vi "Rawdata_Viewer.vi"() -> ()   [LabVIEW 2020]
uses:
  ctl/Image_RAW_Bayer_Pattern.ctl
  ctl/Image_Configuration.ctl
panel:
  out "Total Frame Num":i64
  in  "stop":bool
  in  "Display":bool
  in  "Frame Index":u32
  out "Image":T1(plugin-control)
  in  "Image Configuration":T2={"Width"=3840, "Height"=2160}
  in  "Bayer Pattern":T3=enum."RGGB (GRBG)"
  in  "RAWdata File Path":path
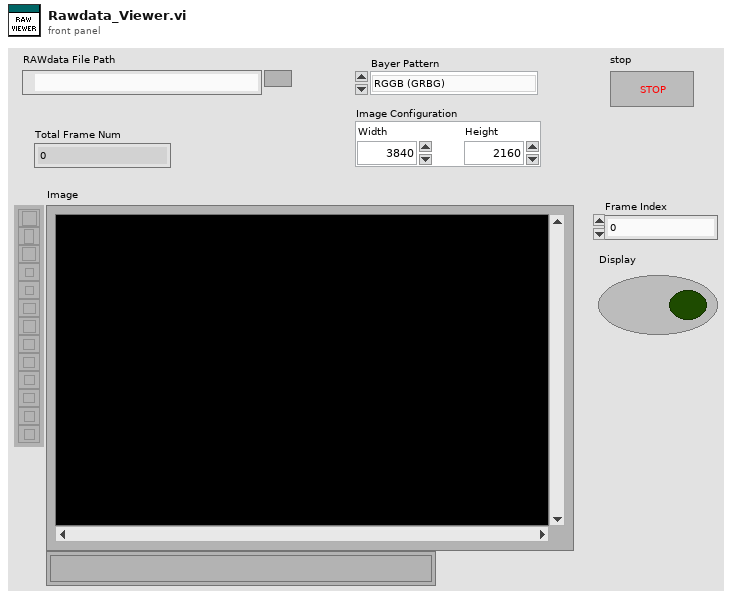
[diagram p1: front panel]
types:
  T1 = typedef "IMAQ Image.ctl" = refnum<image>
  T2 = typedef "Image_Configuration.ctl" = cluster{"Width":i32, "Height":i32}
  T3 = typedef "Image_RAW_Bayer_Pattern.ctl" = enum16{"GBRG (BGGR)", "GRBG (RGGB)", "BGGR (GBRG)", "RGGB (GRBG)", "CRBC (RCCB)"}
  T4 = typedef "Image_Data_Config.ctl" = cluster{"Lines of Image Data":u16, "Bytes per Even Line":u16, "Bytes per Odd Line":u16, "Image Data Type":u8, "Total Image Data Block Size":u32, "Image Data Block Offset":u32}
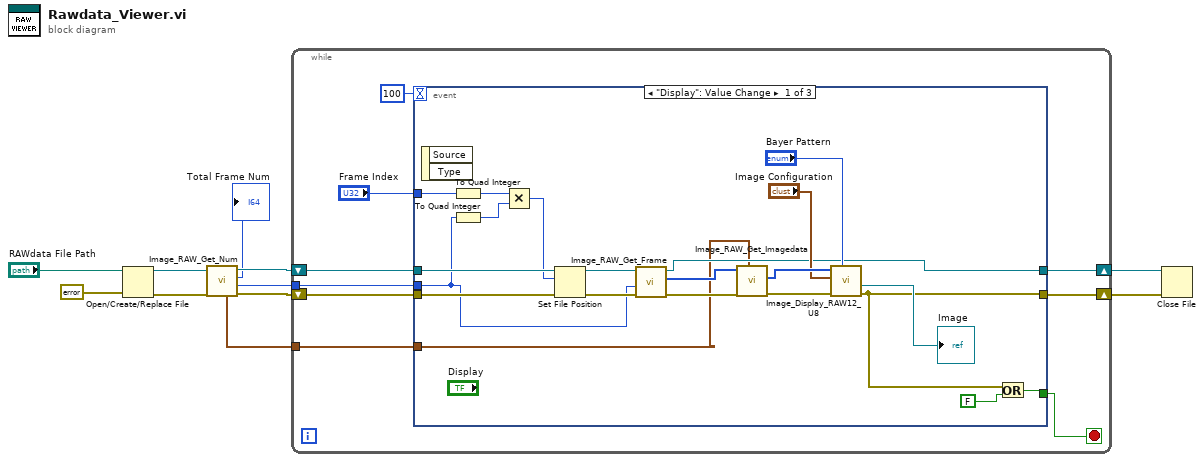
[diagram p0: block diagram]
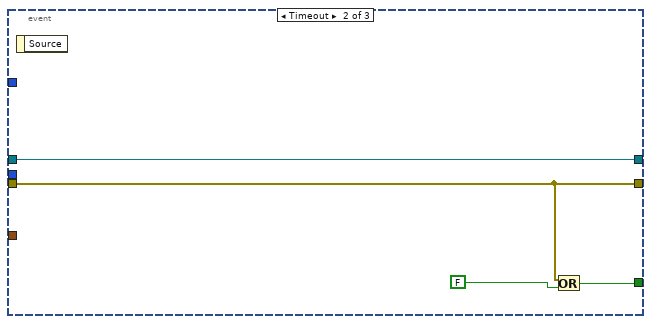
[diagram p2: hidden frame]
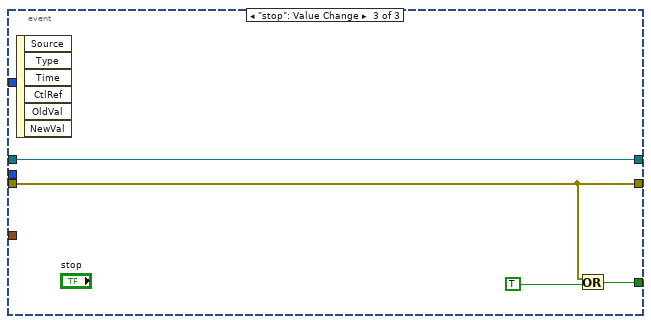
[diagram p3: hidden frame]
diagram:
  n1 = Open/Create/Replace File(file path (use dialog)="RAWdata File Path", error in=errorcluster {"status"=FALSE, "code"=0, "source"=""}) -> (refnum out=w10:refnum<file>, error out=w9:errorcluster)  [unwired: 4 in, 1 out]
  n2 = call "Image_RAW_Get_Num.vi"("error in (no error)"=w9, "RAW refnum In"=w10) -> ("error out"=w5:errorcluster, "Bytes per Frame"=w2:u32, "Total Frame Num"=→"Total Frame Num":i64, "RAW refnum Out"=w6:refnum<file>, "Image Data Config"=w3:T4)  [unwired: 4 in, 1 out]
  n3 = while {
    tunnel: w3 -> [w16]
    tunnel: w2 -> [w14]
    shift-right: [w17] -> w4
    shift-left: w6 -> [w19]
    shift-right: [w20] -> w7
    shift-left: w5 -> [w18]
    stop <- w12 stop-if-true
    n4 = event shown="[0] \"Display\": Value Change" {
      selector: _ -> [_ _ _]
      dyn-events: _ -> [_ _ _]
      timeout: 100 -> [_ _ _]
      tunnel: [w22 w42 w48] -> w20
      tunnel: w19 -> [w37 w45 w49]
      tunnel: w18 -> [w35 w42 w48]
      tunnel: [w30 w45 w49] -> w17
      tunnel: w16 -> [w29 _ _]
      tunnel: "Frame Index" -> [w28 _ _]
      tunnel: w14 -> [w26 _ _]
      tunnel: [w23 w44 w47] -> w12
      event "Display": Value Change {
        n5 = event-data() -> ()  [unwired: 1 in, 2 out]
        n6 = To Quad Integer(1:w28) -> (0:w27:i64)
        n7 = To Quad Integer(1:w26) -> (0:w25:i64)
        n8 = Multiply(x=w27, y=w25) -> (x*y=w36:i64)
        n9 = Set File Position(offset (in bytes) (0)=w36, refnum=w37, error in=w35) -> (refnum out=w34:refnum<file>, error out=w33:errorcluster)  [unwired: 1 in]
        n10 = call "Image_RAW_Get_Frame.vi"("error in (no error)"=w33, "Bytes per Frame"=w26, "RAW refnum In"=w34) -> ("error out"=w31:errorcluster, "Frame (U8)"=w32:u8[], "RAW refnum Out"=w30:refnum<file>)  [unwired: 6 in]
        n11 = call "Image_RAW_Get_Imagedata.vi"("Image Data Config"=w29, "error in (no error)"=w31, "Frame (U8)"=w32) -> ("error out"=w39:errorcluster, "Image Data Payload"=w41:u8[])  [unwired: 7 in]
        n12 = call "Image_Display_RAW12_U8.vi"("Bayer Pattern"="Bayer Pattern", "error in (no error)"=w39, "Image Configuration"="Image Configuration", "RAW12 Frame (U8)"=w41) -> ("error out"=w22:errorcluster, "Image"=→"Image":T1)  [unwired: 4 in, 2 out]
        n13 = Or(x=w22, y=FALSE) -> (x .or. y?=w23:bool)
      }
      event Timeout {
        n14 = event-data() -> ()  [unwired: 1 in, 1 out]
        n15 = Or(x=w42, y=FALSE) -> (x .or. y?=w44:bool)
      }
      event "stop": Value Change {
        n16 = event-data() -> ()  [unwired: 1 in, 6 out]
        n17 = Or(x=w48, y=TRUE) -> (x .or. y?=w47:bool)
      }
    }
  }
  n18 = Close File(refnum=w4, error in=w7) -> ()  [unwired: 2 out]
